vi "gaussian_filter_kernel.vi"(10 "sigma":dbl, 11 "size":i32) -> (3 "Gaussian":dbl[][](array[numeric]))   [LabVIEW 2016]
doc: "Produces 2D Gaussian Kernel for use in spatial filtering. Kernel will be an array of 'Size' x 'Size' with Gaussian sigma of 'sigma'."
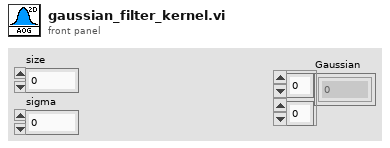
[diagram p1: front panel]
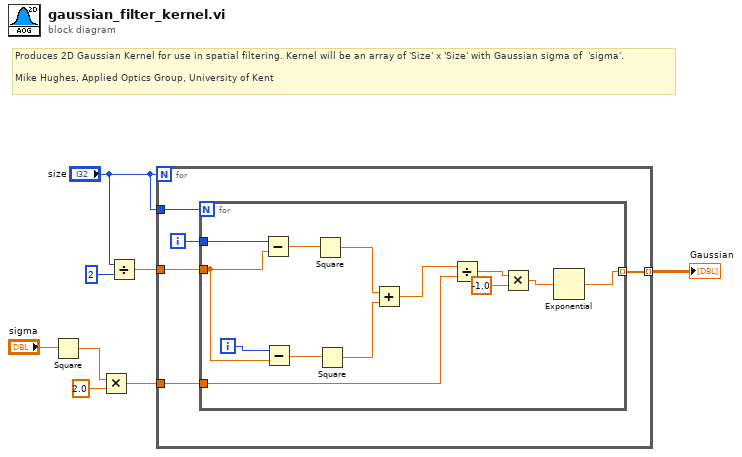
[diagram p0: block diagram]
diagram:
  # "Produces 2D Gaussian Kernel for use in spatial filtering. Kernel will be an array of 'Size' x 'Size' with Gaussian sigma of  'sigma'.\n\nMike Hughes, Applied Optics Group, University of Kent"
  n1 = Square(x="sigma") -> (x^2=w3:dbl)
  n2 = Multiply(x=w3, y=2.0) -> (x*y=w2:dbl)
  n3 = Divide(x="size", y=2) -> (x/y=w6:dbl)
  n4 = for {
    N: "size" -> [_]
    tunnel: "size" -> [w13]
    tunnel: w6 -> [w11]
    tunnel: w2 -> [w10]
    tunnel: [w9] -> w1 mode=indexing
    i -> [w12]
    n5 = for {
      N: w13 -> [_]
      tunnel: w12 -> [w26]
      tunnel: w11 -> [w24]
      tunnel: w10 -> [w18]
      tunnel: [w14] -> w9 mode=indexing
      i -> [w25]
      n6 = Subtract(x=w26, y=w24) -> (x-y=w23:dbl)
      n7 = Subtract(x=w25, y=w24) -> (x-y=w22:dbl)
      n8 = Square(x=w23) -> (x^2=w21:dbl)
      n9 = Square(x=w22) -> (x^2=w20:dbl)
      n10 = Add(x=w21, y=w20) -> (x+y=w19:dbl)
      n11 = Divide(x=w19, y=w18) -> (x/y=w17:dbl)
      n12 = Multiply(x=w17, y=-1.0) -> (x*y=w15:dbl)
      n13 = Exponential(1:w15) -> (0:w14:dbl)
    }
  }
  "Gaussian" <- w1
